vi "Set Power.vi"(7 "Correlation ID":u32, 8 "error in (no error)":errorcluster, 9 "Power":dbl, 11 "Thorlabs Polarizer in":refnum<class "Thorlabs Polarizer.lvclass">) -> (0 "error out":errorcluster, 3 "Thorlabs Polarizer out":refnum<class "Thorlabs Polarizer.lvclass">)   [LabVIEW 2023, in "Thorlabs Polarizer.lvlib" / "Thorlabs Polarizer.lvclass"]
uses:
  Thorlabs Polarizer.lvclass
  Thorlabs Polarizer.lvclass/Thorlabs Polarizer.ctl
  Thorlabs Polarizer.lvlib
  Laser/Laser.lvclass
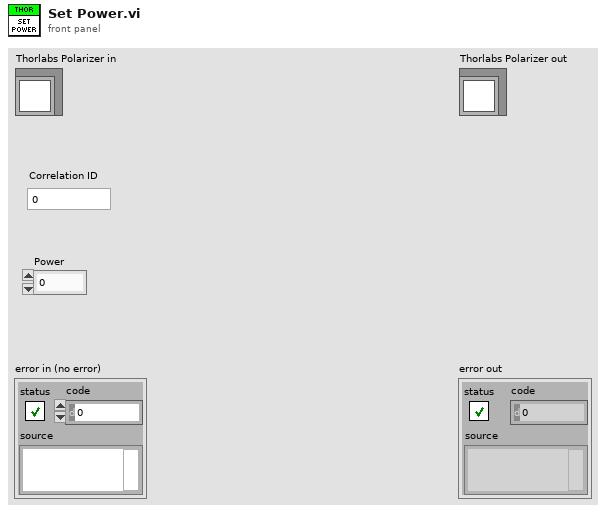
[diagram p1: front panel]
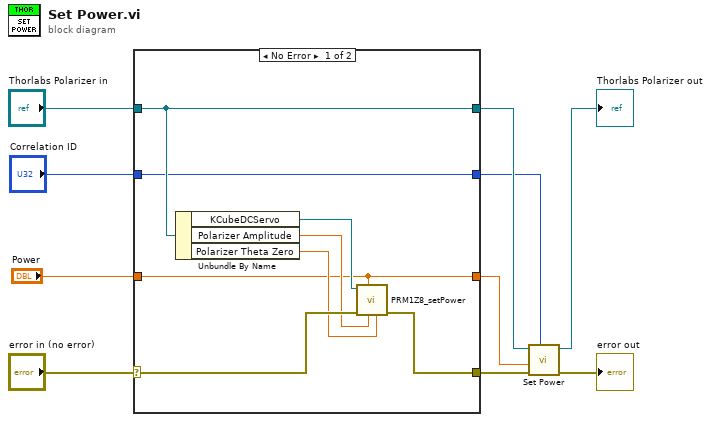
[diagram p0: block diagram]
diagram:
  n1 = case shown="No Error" "error in (no error)" {
    selector: "error in (no error)" -> [w18 w22]
    tunnel: [w17 w22] -> w7
    tunnel: [w14 w21] -> w5
    tunnel: "Thorlabs Polarizer in" -> [w14 w21]
    tunnel: "Power" -> [w12 w20]
    tunnel: [w12 w20] -> w3
    tunnel: "Correlation ID" -> [w11 w19]
    tunnel: [w11 w19] -> w1
    frame No Error {
      n2 = Unbundle By Name(w14) -> ("KCubeDCServo"=w13:refnum<k24>, "Polarizer Amplitude"=w16:dbl, "Polarizer Theta Zero"=w15:dbl)
      n3 = call "PRM1Z8_setPower.vi"("zero angle"=w15, "max power"=w16, "Target Power"=w12, "error in (no error)"=w18, "reference"=w13) -> ("error out"=w17:errorcluster)  [unwired: 5 in, 1 out]
    }
    frame Error {
    }
  }
  n4 = call-parent "Set Power.vi"("Correlation ID"=w1, "error in (no error)"=w7, "Power"=w3, "Laser Quantum in"=w5) -> ("error out"=→"error out":errorcluster, "Laser Quantum out"=→"Thorlabs Polarizer out":refnum<class "Thorlabs Polarizer.lvclass">)  [unwired: 6 in]
